vi "Main.vi"(11 "Module Admin":refnum<class "Delacor_lib_QMH_Module Admin.lvclass">) -> ()   [LabVIEW 2020, in "Peek Window.lvlib"]
doc: "This template is based off of the Queued Message Handler design pattern and the Queued Message Handler project template that ships with LabVIEW.\n\nThe main difference is that the queue is private to this module and communication between modules is performed via Broadcast and Request events.\n\nRequest events are wrapped in public API methods and are handled in the Event Handling Loop (EHL) of this VI. Any module can register for Broadcast events sent by this module. The EHL generates messages based on user interface actions.\n\nThe Message Handling Loop (MHL) processes messages generated by the EHL, or by other messages. The messages are string values, so new messages can be added easily to the Message Cases case structure in the MHL. Each message cluster can also provide an optional value for Message Data, which is a variant that can be converted to whatever message-specific data is required.\n_____\nBased on Delacor QMH Project Template 5.0.0.82."
uses:
  Peek Window.lvlib
  <vilib>/Delacor/Delacor QMH/Libraries/Module Admin_class/Delacor_lib_QMH_Module Admin.lvclass
  MHL Data Cluster.ctl
  Open Diagram Argument--cluster.ctl
  EHL Data Cluster.ctl
  Active VI Cluster.ctl
  <vilib>/Delacor/Delacor QMH/Libraries/Message Queue_class/Delacor_lib_QMH_Message Queue.lvclass/Delacor_lib_QMH_Message Queue.ctl
  Stop Argument--cluster.ctl
  <vilib>/Delacor/Delacor QMH/Libraries/Module Admin_class/Delacor_lib_QMH_Module Admin.lvclass/Delacor_lib_QMH_Module Admin.ctl
  Invalid Selection Argument--cluster.ctl
  <vilib>/Delacor/Delacor QMH/Libraries/Message Queue_class/Delacor_lib_QMH_Enqueue Message (Single).vi
  <vilib>/Delacor/Delacor QMH/Libraries/Module Admin_class/Delacor_lib_QMH_Get External Launch.vi
  <vilib>/Utility/error.llb/Error Cluster From Error Code.vi
  <vilib>/ErrorRing/Error Ring.xnode
  <vilib>/Delacor/Delacor QMH/Libraries/Message Queue_class/Delacor_lib_QMH_Message Queue.lvclass
panel:
  in  "File Open":bool
  in  "Previous":bool
  in  "Pin?":bool
  out "Application":string
  in  "Simulate MHL Error":bool
  in  "Simulate EHL Error":bool
  out "error out":errorcluster
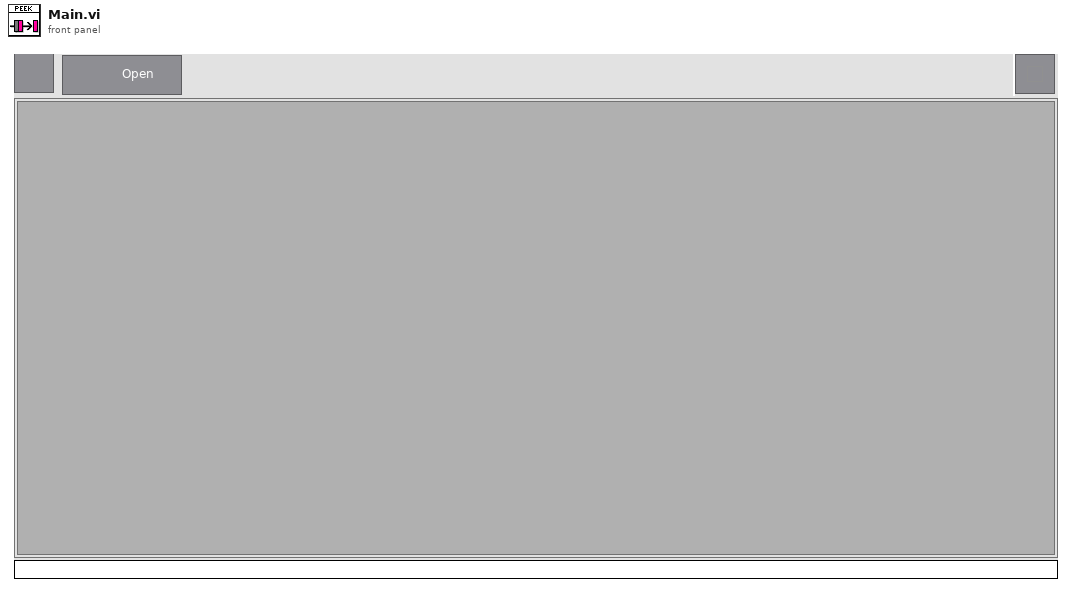
[diagram p1: front panel]
types:
  T1 = typedef "Peek Window.lvlib/EHL Data Cluster.ctl" = cluster{"VI Inserted":string, "Active VI":T2}
  T2 = typedef "Peek Window.lvlib/Active VI Cluster.ctl" = cluster{"App Refnum":refnum<vi>, "VIName":string}
  T3 = typedef "Peek Window.lvlib/MHL Data Cluster.ctl" = cluster{"SubPanel":refnum<vi>, "Call Chain":string[], "Active VI":T4}
  T4 = typedef "Peek Window.lvlib/Open Diagram Argument--cluster.ctl" = cluster{"VI Name":string, "Owning VI Name":string, "App Refnum":refnum<vi>}
  T5 = typedef "Peek Window.lvlib/Request Events--cluster.ctl" = cluster{"Stop Module":refnum<user-event>, "Show Panel":refnum<user-event>, "Hide Panel":refnum<user-event>, "Get Module Execution Status":refnum<user-event>, "Show Diagram":refnum<user-event>, "Open Diagram":refnum<user-event>, "Invalid Selection":refnum<user-event>}
  T6 = enum32{"invalid lock state", "Not Locked", "Locked (No Password)", "Password-protected"}
  T7 = typedef "Peek Window.lvlib/Stop Argument--cluster.ctl" = cluster{"Origin":string, "Exit via Stop Module Req?":bool, "Wait for Module to stop?":bool}
  T8 = typedef "Peek Window.lvlib/Invalid Selection Argument--cluster.ctl" = cluster{"Active VI":string}
  T9 = enum32{"Invalid", "Standard", "Closed", "Hidden", "Minimized", "Maximized"}
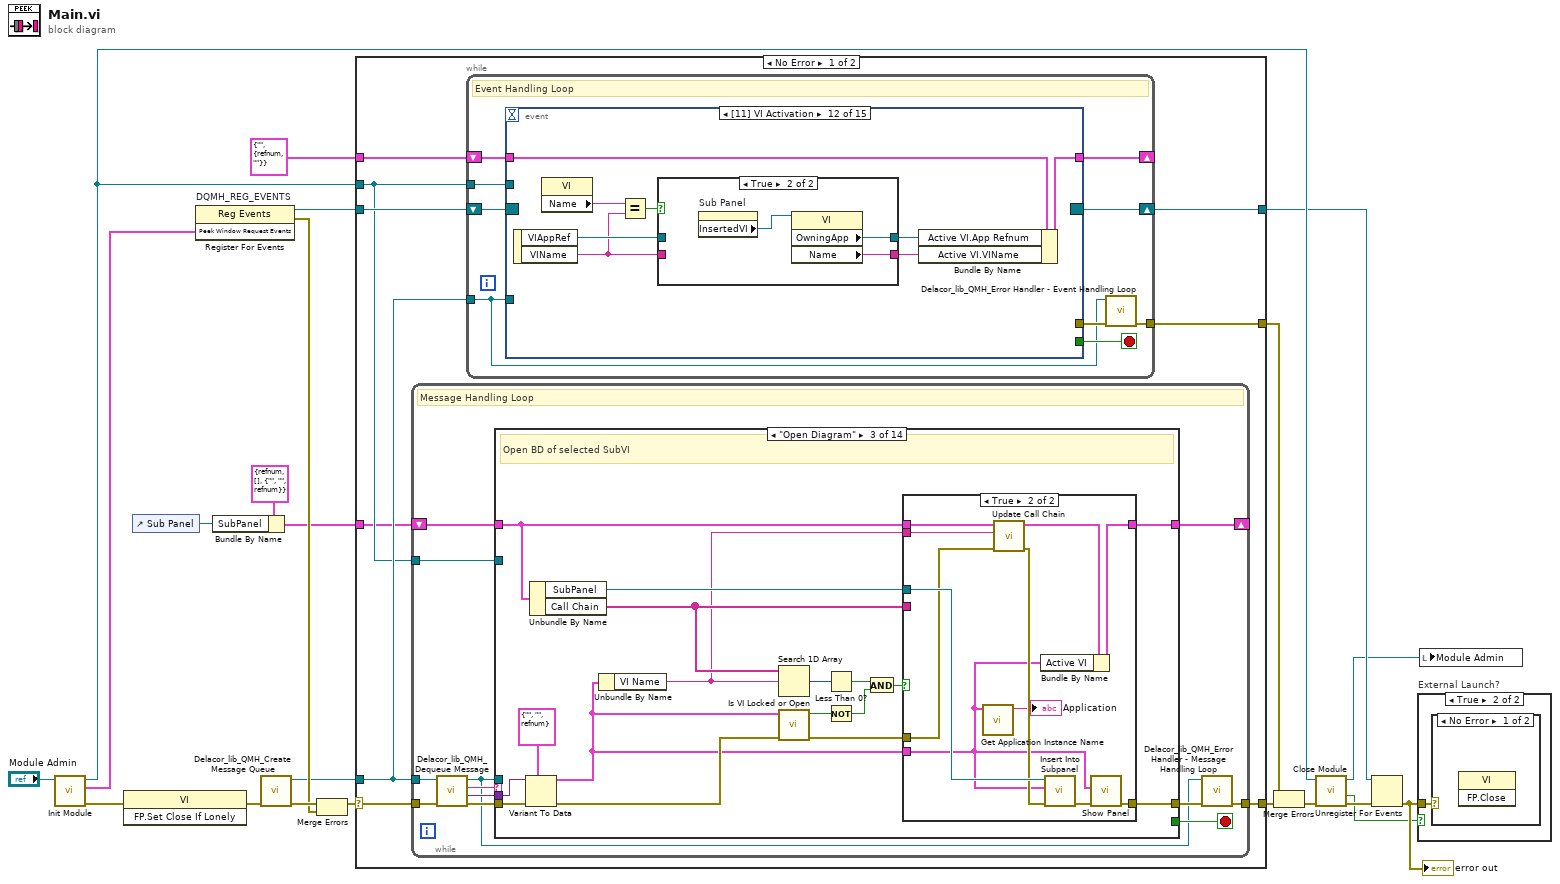
[diagram p0: block diagram]
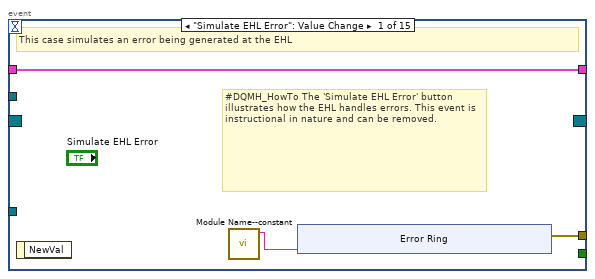
[diagram p2: hidden frame]
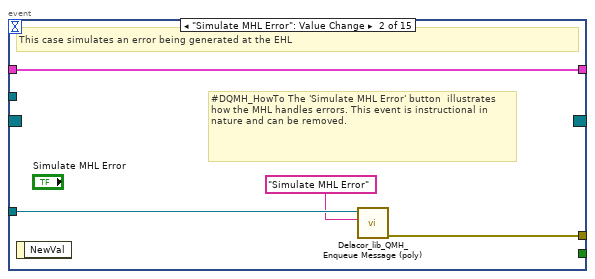
[diagram p3: hidden frame]
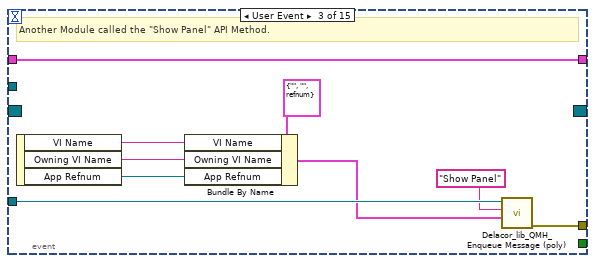
[diagram p4: hidden frame]
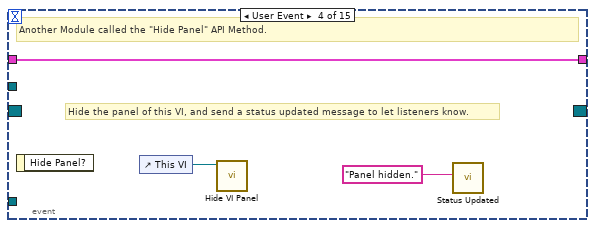
[diagram p5: hidden frame]
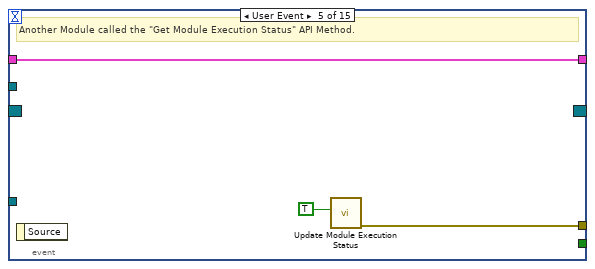
[diagram p6: hidden frame]
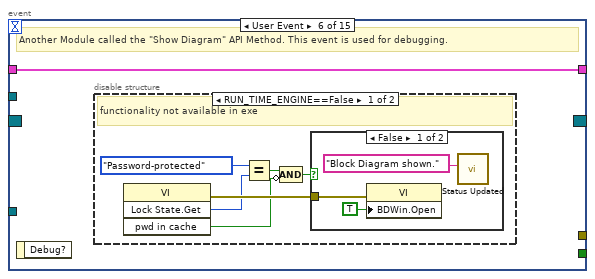
[diagram p7: hidden frame]
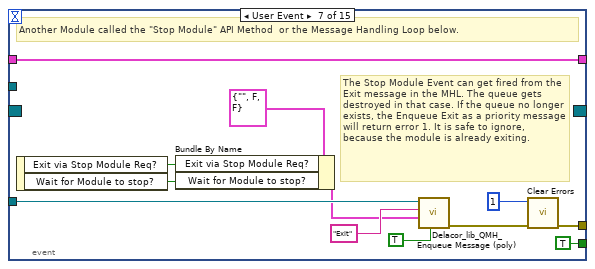
[diagram p10: hidden frame]
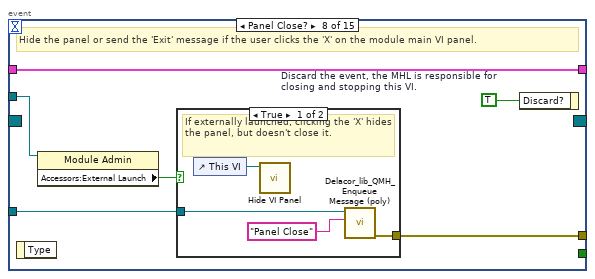
[diagram p11: hidden frame]
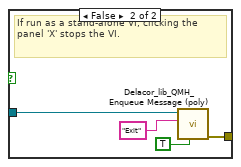
[diagram p12: hidden frame]
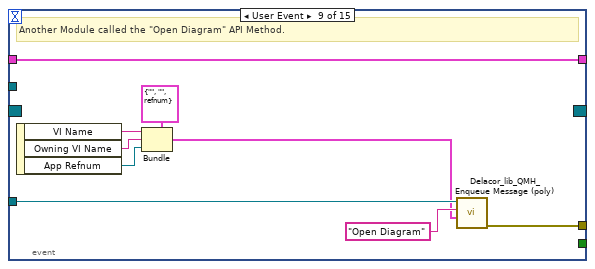
[diagram p13: hidden frame]
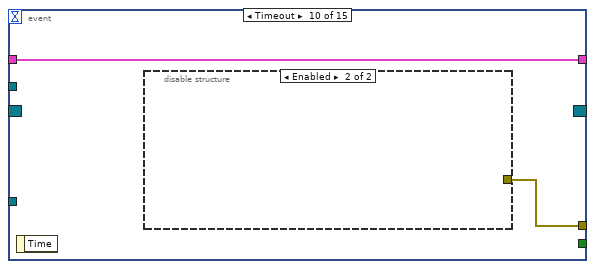
[diagram p14: hidden frame]
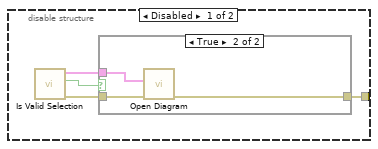
[diagram p15: hidden frame]
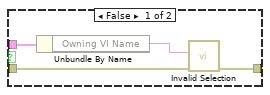
[diagram p16: hidden frame]
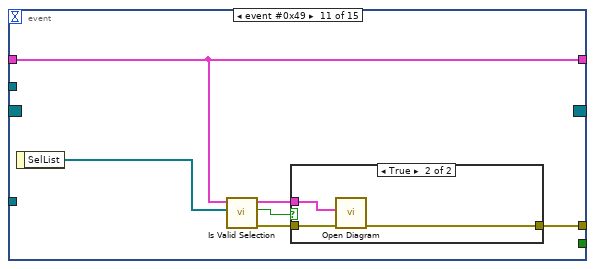
[diagram p17: hidden frame]
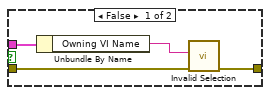
[diagram p18: hidden frame]
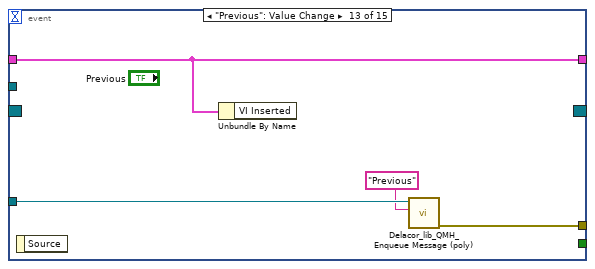
[diagram p20: hidden frame]
diagram:
  n1 = call "Init Module.vi"("Singleton Module Admin in"="Module Admin") -> ("error out"=w2:errorcluster, "Peek Window Request Events"=w11:T5, "Singleton Module Admin out"=w14:refnum<class "Delacor_lib_QMH_Module Admin.lvclass">)  [unwired: 8 in]
  n2 = invoke class="VI" method="FP.Set Close If Lonely"(error in=w2) -> (error out=w1:errorcluster)  [unwired: 2 in, 2 out]
  n3 = control-ref of="Sub Panel"() -> (w4:refnum<vi>)
  n4 = register-events "DQMH_REG_EVENTS"(w11) -> (reference out=w12:refnum<event-registration>, error out=w15:errorcluster)  [unwired: 2 in]
  n5 = Bundle By Name(cluster=T3 {"SubPanel"=refnum, "Call Chain"=[], "Active VI"={"VI Name"="", "Owning VI Name"="", "App Refnum"=refnum}} ("Data Cluster"), "SubPanel"=w4) -> (w5:T3)
  n6 = call <vilib>:"Delacor_lib_QMH_Create Message Queue.vi"("error in (no error)"=w1) -> ("error out"=w17:errorcluster, "Message Queue"=w10:refnum<class "Delacor_lib_QMH_Message Queue.lvclass">)  [unwired: 9 in]
  n7 = Merge Errors(w17, w15) -> (w16:errorcluster)
  n8 = case shown="No Error" w16 {
    selector: w16 -> [w29 w392]
    tunnel: [w31 w391] -> w22
    tunnel: [w28 w397] -> w13
    tunnel: w12 -> [w27 w397]
    tunnel: w10 -> [w26 w390]
    tunnel: [w30 _] -> w20
    tunnel: w14 -> [w25 w393]
    tunnel: w5 -> [w24 _]
    tunnel: T1 {"VI Inserted"="", "Active VI"={"App Refnum"=refnum, "VIName"=""}} ("Data") -> [w23 _]
    frame No Error {
      n9 = while {
        tunnel: w26 -> [w172]
        shift-right: [w169] -> _
        shift-left: w24 -> [w176]
        tunnel: w29 -> [w179]
        tunnel: [w177] -> w31
        tunnel: w25 -> [w170]
        stop <- w175 stop-if-true
        # "Message Handling Loop"
        n10 = call-dynamic "Delacor_lib_QMH_Dequeue Message.vi"("error in (no error)"=w179, "Message Queue in"=w172) -> ("error out"=w178:errorcluster, "Message Data"=w173:variant, "Message"=w174:string, "Message Queue out"=w171:refnum<class "Delacor_lib_QMH_Message Queue.lvclass">)  [unwired: 6 in]
        n11 = case "DQMH_MESSAGE_CASES" shown="\"Open Diagram\"" w174 {
          selector: w174 -> [_ _ _ _ _ _ _ _ _ _ _ _ _ w377]
          tunnel: w171 -> [_ _ _ _ _ _ _ _ _ _ _ w347 w369 _]
          tunnel: w178 -> [w195 w199 w216 w233 w262 w279 w302 w317 w329 w331 w336 w354 w375 w379]
          tunnel: [w193 w199 w213 w238 w257 w280 w302 w308 w328 w331 w335 w350 w372 w380] -> w180
          tunnel: w176 -> [w184 w198 w210 w236 w267 w269 w301 w304 w327 w330 w333 w349 w368 w378]
          tunnel: [w184 w198 w211 w237 w266 w270 w300 w303 w327 w330 w333 w349 w368 w378] -> w169
          tunnel: [_ _ _ _ _ _ _ _ _ _ _ _ w367 _] -> w175
          tunnel: w173 -> [_ _ w215 _ _ w276 _ w316 _ _ _ w348 w366 _]
          tunnel: w170 -> [w185 _ _ _ _ _ _ _ _ _ _ w346 w361 _]
          frame "Initialize" {
            # "#CodeNeeded - Initialize the appearance of the front panel."
            # "#CodeNeeded - Initialize your state data here."
            # "Initialize - Any operation that needs to be done before the module can receive messages. Synchronize Caller Events.vi will inform Start Module.vi that the module has launched and is ready to receive messages. Module Did Init.vi will broadcast that the module initialized."
            n12 = call "Synchronize Caller Events.vi"("error in (no error)"=w195, "Singleton Module Admin in"=w185) -> ("error out"=w194:errorcluster, "Singleton Module Admin out"=w181:refnum<class "Delacor_lib_QMH_Module Admin.lvclass">)  [unwired: 8 in]
            n13 = property on="Property Node" class="Module Admin"(reference=w181) -> ("Accessors:External Launch"=w189:bool)  [unwired: 1 in, 2 out]
            n14 = Select(t=T9."Hidden" ("State"), s=w189, f=T9."Standard" ("State")) -> (s? t:f=w186:T9)
            n15 = call "Module Name--constant.vi"() -> ("Module Name"=w192:string)  [unwired: 11 in]
            n16 = property on="Property Node" class="VI"("Front Panel.Title"=w192) -> (reference out=w191:refnum<vi>, error out=w197:errorcluster)  [unwired: 2 in]
            n17 = call "Module Name--constant.vi"() -> ("Module Name"=w182:string)  [unwired: 11 in]
            n18 = invoke on="Invoke Node" class="VI" method="FP.Open"(reference=w191, error in=w197, "State"=w186) -> (reference out=w190:refnum<vi>, error out=w196:errorcluster)  [unwired: 2 in, 3 out]
            n19 = call "Module Did Init.vi"("error in (no error)"=w194, "Initialized?"=TRUE, "Origin"=w182) -> ("error out"=w193:errorcluster)  [unwired: 8 in]
            n20 = invoke on="Invoke Node" class="VI" method="FP.Center"(reference=w190, error in=w196) -> ()  [unwired: 1 in, 3 out]
          }
          frame "--- Module Specific ---" {
            # "Separator -- The following cases handle messages specific to this Module."
          }
          frame "Open Diagram" {
            # "Open BD of selected SubVI"
            n21 = Variant To Data(error in=w216, type=T4 {"VI Name"="", "Owning VI Name"="", "App Refnum"=refnum} ("Open Diagram Argument"), Variant=w215) -> (data=w200:T4, error out=w204:errorcluster)
            n22 = Unbundle By Name(w210) -> ("SubPanel"=w208:refnum<vi>, "Call Chain"=w209:string[])
            n23 = Unbundle By Name(w200) -> ("VI Name"=w201:string)
            n24 = Search 1D Array(1D array=w209, element=w201) -> (index of element=w212:i32)  [unwired: 1 in]
            n25 = call "Is VI Locked or Open.vi"("Error In"=w204, "VI Info"=w200) -> ("Error Out"=w203:errorcluster, "Locked or Open?"=w206:bool)  [unwired: 8 in]
            n26 = Less Than 0?(x=w212) -> (x < 0?=w207:bool)
            n27 = Not(x=w206) -> (.not. x?=w205:bool)
            n28 = And(x=w207, y=w205) -> (x .and. y?=w202:bool)
            n29 = case shown="True" w202 {
              tunnel: [w218 w224] -> w213
              tunnel: w203 -> [w218 w227]
              tunnel: w201 -> [_ w223]
              tunnel: [w217 w221] -> w211
              tunnel: w210 -> [w217 w228]
              tunnel: w209 -> [_ _]
              tunnel: w208 -> [_ w229]
              tunnel: w200 -> [_ w219]
              frame False {
              }
              frame True {
                n30 = call "Get Application Instance Name.vi"("Active Components"=w219) -> ("Name"=→"Application":string)  [unwired: 10 in]
                n31 = call "Update Call Chain.vi"("error in (no error)"=w227, "VI Name"=w223, "Data Cluster in"=w228) -> ("error out"=w226:errorcluster, "Data Cluster out"=w222:T3)  [unwired: 7 in]
                n32 = Bundle By Name(cluster=w222, "Active VI"=w219) -> (w221:T3)
                n33 = call "Insert Into Subpanel.vi"("error in (no error)"=w226, "Active Components"=w219, "SubPanel in"=w229) -> ("error out"=w225:errorcluster)  [unwired: 7 in, 1 out]
                n34 = call "Show Panel.vi"("error in (no error)"=w225, "Open Diagram Argument"=w219) -> ("error out"=w224:errorcluster)  [unwired: 9 in]
              }
            }
          }
          frame "Previous" {
            # "Open BD of previous SubVI"
            n35 = Unbundle By Name(w236) -> ("Call Chain"=w235:string[], "Active VI"=w231:T4, "SubPanel"=w230:refnum<vi>)
            n36 = Delete From Array(array=w235) -> (array with subset deleted=w234:string[])  [unwired: 2 in, 1 out]
            n37 = Empty Array?(array=w234) -> (empty?=w232:bool)
            n38 = case shown="False" w232 {
              tunnel: [w243 w250] -> w238
              tunnel: [w247 w251] -> w237
              tunnel: w236 -> [w249 w251]
              tunnel: w234 -> [w246 _]
              tunnel: w233 -> [w248 w250]
              tunnel: w230 -> [w239 _]
              tunnel: w231 -> [w241 _]
              frame False {
                n39 = Delete From Array "Replace showing VI\nwith most recent in\ncall chain"(array=w246) -> (deleted portion=w242:string)  [unwired: 2 in, 1 out]
                n40 = Bundle By Name(cluster=w241, "VI Name"=w242) -> (w240:T4)
                n41 = control-ref of="This VI"() -> (w245:refnum<vi>)
                n42 = Bundle By Name(cluster=w249, "Call Chain"=w246) -> (w247:T3)
                n43 = call "Insert Into Subpanel.vi"("error in (no error)"=w248, "Active Components"=w240, "SubPanel in"=w239) -> ("error out"=w244:errorcluster)  [unwired: 7 in, 1 out]
                n44 = call "Position Peek Window.vi"("Error In"=w244, "Subpanel"=w239, "Active Components"=w240, "PeekVI Reference"=w245) -> ("error out"=w243:errorcluster)  [unwired: 7 in]
              }
              frame True {
              }
            }
          }
          frame "File Open" {
            # "Open VI in Current Window"
            n45 = Unbundle By Name(w267) -> ("Active VI.App Refnum"=w252:refnum<vi>, "Call Chain"=w264:string[], "SubPanel"=w261:refnum<vi>)
            n46 = invoke class="SubPnl" method="Remove VI"(reference=w261, error in=w262) -> (error out=w256:errorcluster)  [unwired: 1 in, 2 out]
            n47 = property class="VI"(error in=w256, "FP.State"=T9."Hidden" ("Front Panel Window:State")) -> (error out=w255:errorcluster)  [unwired: 1 in, 1 out]
            n48 = Delete From Array(array=w264) -> (deleted portion=w263:string)  [unwired: 2 in, 1 out]
            n49 = Open VI Reference(application reference (local)=w252, vi path=w263, error in (no error)=w255) -> (vi reference=w259:refnum<vi>, error out=w260:errorcluster)  [unwired: 3 in]
            n50 = Bundle By Name(cluster=w267, "Call Chain"=string[] []) -> (w266:T3)
            n51 = property class="VI"(reference=w259, error in=w260, "BDWin.Open"=TRUE ("Block Diagram Window:Open"), "FP.State"=T9."Minimized" ("Front Panel Window:State")) -> (error out=w257:errorcluster)  [unwired: 1 out]
          }
          frame "Show Panel" {
            n52 = Variant To Data(error in=w279, type=T4 {"VI Name"="", "Owning VI Name"="", "App Refnum"=refnum} ("Open Diagram Argument"), Variant=w276) -> (data=w268:T4, error out=w277:errorcluster)
            n53 = Bundle By Name(cluster=w269, "Active VI"=w268) -> (w270:T3)
            n54 = Unbundle By Name(w270) -> ("Call Chain"=w273:string[], "SubPanel"=w271:refnum<vi>)
            n55 = control-ref of="This VI"() -> (w275:refnum<vi>)
            n56 = Empty Array?(array=w273) -> (empty?=w272:bool)
            n57 = case shown="False" w272 {
              tunnel: [w286 w298] -> w280
              tunnel: w277 -> [w287 w298]
              tunnel: "Pin?" -> [w285 _]
              tunnel: w268 -> [w283 _]
              tunnel: w275 -> [w284 _]
              tunnel: w273 -> [w282 _]
              tunnel: w271 -> [w281 _]
              frame False {
                # "Call Chain not empty"
                n58 = case shown="False" w285 {
                  tunnel: w287 -> [w294 w297]
                  tunnel: [w295 w297] -> w286
                  tunnel: w284 -> [w293 _]
                  tunnel: w283 -> [w289 _]
                  tunnel: w282 -> [w291 _]
                  tunnel: w281 -> [w288 _]
                  frame False {
                    # "Not pinned"
                    n59 = Delete From Array "Replace showing VI\nwith most recent in\ncall chain"(array=w291) -> (deleted portion=w292:string)  [unwired: 2 in, 1 out]
                    n60 = Bundle By Name(cluster=w289, "VI Name"=w292) -> (w290:T4)
                    n61 = call "Position Peek Window.vi"("Error In"=w294, "Subpanel"=w288, "Active Components"=w290, "PeekVI Reference"=w293) -> ("error out"=w295:errorcluster)  [unwired: 7 in]
                  }
                  frame True {
                    # "Pinned"
                    n62 = property class="VI"("FP.State"=T9."Standard" ("Front Panel Window:State")) -> ()  [unwired: 2 in, 2 out]
                  }
                }
              }
              frame True {
                # "Nothing in Call Chain"
              }
            }
          }
          frame "Panel Close" {
            n63 = Bundle By Name(cluster=w301, "Call Chain"=string[] []) -> (w300:T3)
          }
          frame "Invalid Selection" {
            n64 = Variant To Data(error in=w317, type=T8 {"Active VI"=""} ("Invalid Selection Argument"), Variant=w316) -> (data=w314:T8, error out=w309:errorcluster)
            n65 = Unbundle By Name(w304) -> ("Call Chain"=w313:string[])
            n66 = property class="VI"() -> ("Name"=w312:string)  [unwired: 2 in, 2 out]
            n67 = Unbundle By Name(w314) -> ("Active VI"=w310:string)
            n68 = Build Array (concatenate)(w313, w312, "VI Hierarchy") -> (w311:string[])
            n69 = Search 1D Array(1D array=w311, element=w310) -> (index of element=w307:i32)  [unwired: 1 in]
            n70 = Less Than 0?(x=w307) -> (x < 0?=w306:bool)
            n71 = case shown="True" w306 {
              tunnel: w309 -> [w319 w321]
              tunnel: [w319 w320] -> w308
              tunnel: w304 -> [w318 w323]
              tunnel: [w318 w325] -> w303
              frame False {
              }
              frame True {
                n72 = Unbundle By Name(w323) -> ("SubPanel"=w322:refnum<vi>)
                n73 = invoke class="SubPnl" method="Remove VI"(reference=w322, error in=w321) -> (error out=w320:errorcluster)  [unwired: 1 in, 2 out]
                n74 = property class="VI"("FP.State"=T9."Hidden" ("Front Panel Window:State")) -> ()  [unwired: 2 in, 2 out]
                n75 = Bundle By Name(cluster=w323, "Call Chain"=string[] []) -> (w325:T3)
              }
            }
          }
          frame "---Copy This Frame---" {
            # "Duplicate this frame when creating new messages.  Change this comment in the duplicated frame to describe this message."
            n76 = Merge Errors(w329) -> (w328:errorcluster)
          }
          frame "--- Exit and Error Handling---" {
            # "Separator - The following cases handle errors and exit messages."
          }
          frame "Simulate MHL Error" {
            # "#DQMH_HowTo The 'Simulate MHL Error' button  illustrates how the MHL handles errors. This event is instructional in nature and can be removed."
            # "Simulate an error occurring at the MHL"
            n77 = call "Module Name--constant.vi"() -> ("Module Name"=w332:string)  [unwired: 11 in]
            n78 = xnode "Error Ring"("parameter 0"=w332) -> ("error out"=w334:errorcluster)
            n79 = Merge Errors(w336, w334) -> (w335:errorcluster)
          }
          frame "Error" {
            # "#CodeRecommended - If you ever change the name of this \"Error\" message, you'll need to update the name in the Check Loop Error.vi as well."
            # "#CodeRecommended - If the module is running in standalone mode (External Launch = FALSE), this code will pop up an error dialog and call the 'Exit' message if an error occurs. Add more fine-grained error handling here."
            # "Error - Check the error message data and respond accordingly. This message is sent by the \"Error Handler\" VIs at the end of each loop in this application."
            n80 = property on="Property Node" class="Module Admin"(reference=w346) -> ("Accessors:External Launch"=w345:bool)  [unwired: 1 in, 2 out]
            n81 = Variant To Data(error in=w354, type=errorcluster {"status"=FALSE, "code"=0, "source"=""} ("error constant"), Variant=w348) -> (data=w355:errorcluster, error out=w352:errorcluster)
            n82 = call "Module Name--constant.vi"() -> ("Module Name"=w344:string)  [unwired: 11 in]
            n83 = call "Error Reported.vi"("Additional Information"=w344, "Error"=w355) -> ()  [unwired: 9 in, 1 out]
            n84 = case shown="False" w345 {
              tunnel: [w360 _] -> w351
              tunnel: w347 -> [w358 _]
              tunnel: w355 -> [w359 _]
              frame False {
                # "If the module is running standalone, then pop up an error dialog and call the \"Exit\" message."
                n85 = call <vilib>:"Simple Error Handler.vi"("error in (no error)"=w359) -> ()  [unwired: 4 in, 5 out]
                n86 = call-poly <vilib>:"Delacor_lib_QMH_Enqueue Message (poly).vi"("Priority Message? (F)"=TRUE, "Message"="Exit", "Message Queue in"=w358) -> ("error out"=w360:errorcluster)  [unwired: 7 in, 1 out]
              }
              frame True {
                # "If the module was launched externally, calling the Error Reported broadcast VI is the only action performed by the \"Error\" message. The module's caller can then process the error appropriately."
              }
            }
            n87 = Merge Errors(w352, w351) -> (w350:errorcluster)
            n88 = local write "error out"(w350) -> ()
          }
          frame "Exit" {
            w365 = 91  # 91: not all Exit messages will have an argument
            w367 = TRUE  # Stop the VI
            # "Release the message queue reference"
            # "#CodeNeeded - Add any required cleanup code here"
            # "Exit - Exit the application."
            n89 = Variant To Data(error in=w375, type=T7 {"Origin"="", "Exit via Stop Module Req?"=FALSE, "Wait for Module to stop?"=FALSE} ("Stop Argument"), Variant=w366) -> (data=w363:T7, error out=w371:errorcluster)
            n90 = call <vilib>:"Clear Errors.vi"("error in (no error)"=w371, "specific error code to clear (0: all)"=w365) -> ("error out"=w374:errorcluster)  [unwired: 4 in, 1 out]
            n91 = control-ref of="This VI"() -> (w362:refnum<vi>)
            n92 = call-dynamic "Delacor_lib_QMH_Release Message Queue.vi"("error in (no error)"=w374, "Message Queue"=w369) -> ("error out"=w373:errorcluster)  [unwired: 9 in]
            n93 = call "Handle Exit.vi"("Stop Argument"=w363, "Admin in"=w361, "VI reference"=w362) -> ("error out"=w370:errorcluster)  [unwired: 7 in, 1 out]
            n94 = Merge Errors(w373, w370) -> (w372:errorcluster)
          }
          frame Default {
            # "'Default' case only runs if there is a message that isn't defined in any of the other cases.  Output a programming error."
            n95 = call "Module Name--constant.vi"() -> ("Module Name"=w376:string)  [unwired: 11 in]
            n96 = xnode "Error Ring"("parameter 0"=w377, "parameter 1"=w376) -> ("error out"=w381:errorcluster)
            n97 = Merge Errors(w379, w381) -> (w380:errorcluster)
          }
        }
        n98 = call-dynamic "Delacor_lib_QMH_Error Handler - Message Handling Loop.vi"("error in (no error)"=w180, "Message Queue in"=w171) -> ("dup error in"=w177:errorcluster)  [unwired: 8 in, 1 out]
      }
      n99 = while {
        tunnel: w26 -> [w34]
        shift-right: [w37] -> w28
        shift-left: w27 -> [w38]
        tunnel: [w39] -> w30
        tunnel: w25 -> [w35]
        shift-right: [w32] -> _
        shift-left: w23 -> [w33]
        stop <- w36 stop-if-true
        # "Event Handling Loop"
        n100 = event "DQMH_EVENT_MAIN" shown="[11] VI Activation" {
          selector: w38 -> [_ _ _ _ _ _ _ _ _ _ _ _ _ _ _]
          dyn-events: [_ _ _ _ _ _ _ _ _ _ _ _ _ _ _] -> w37
          timeout: _ -> [_ _ _ _ _ _ _ _ _ _ _ _ _ _ _]
          tunnel: [_ _ _ _ _ _ TRUE ("Discard?") _ _ _ _ _ _ _ _] -> w36
          tunnel: w34 -> [_ w53 w62 _ _ _ w87 w95 w114 _ _ _ w157 w160 w167]
          tunnel: [w43 w54 w61 _ w69 _ w90 w97 w109 w115 w131 _ w156 w159 w162] -> w40
          tunnel: w35 -> [_ _ _ _ _ _ _ w94 _ _ _ _ _ _ _]
          tunnel: w33 -> [w41 w51 w63 w64 w67 w70 w80 w92 w108 w116 w129 w147 w154 w161 w168]
          tunnel: [w41 w51 w63 w64 w67 w70 w80 w92 w108 w116 w129 w148 w154 w161 w168] -> w32
          event "Simulate EHL Error": Value Change {
            # "#DQMH_HowTo The 'Simulate EHL Error' button  illustrates how the EHL handles errors. This event is instructional in nature and can be removed."
            # "This case simulates an error being generated at the EHL"
            n101 = event-data() -> ()  [unwired: 1 in, 1 out]
            n102 = call "Module Name--constant.vi"() -> ("Module Name"=w42:string)  [unwired: 11 in]
            n103 = xnode "Error Ring"("parameter 0"=w42) -> ("error out"=w43:errorcluster)
          }
          event "Simulate MHL Error": Value Change {
            # "#DQMH_HowTo The 'Simulate MHL Error' button  illustrates how the MHL handles errors. This event is instructional in nature and can be removed."
            # "This case simulates an error being generated at the EHL"
            n104 = event-data() -> ()  [unwired: 1 in, 1 out]
            n105 = call-poly <vilib>:"Delacor_lib_QMH_Enqueue Message (poly).vi"("Message"="Simulate MHL Error", "Message Queue in"=w53) -> ("error out"=w54:errorcluster)  [unwired: 8 in, 1 out]
          }
          event User Event {
            # "Another Module called the \"Show Panel\" API Method."
            n106 = event-data() -> ("VI Name"=w58:string, "Owning VI Name"=w56:string, "App Refnum"=w55:refnum<vi>)  [unwired: 1 in]
            n107 = Bundle By Name(cluster=T4 {"VI Name"="", "Owning VI Name"="", "App Refnum"=refnum} ("Open Diagram Argument"), "VI Name"=w58, "Owning VI Name"=w56, "App Refnum"=w55) -> (w57:T4)
            n108 = call-poly <vilib>:"Delacor_lib_QMH_Enqueue Message (poly).vi"("Message Data"=w57, "Message"="Show Panel", "Message Queue in"=w62) -> ("error out"=w61:errorcluster)  [unwired: 7 in, 1 out]
          }
          event User Event {
            # "Hide the panel of this VI, and send a status updated message to let listeners know."
            # "Another Module called the \"Hide Panel\" API Method."
            n109 = event-data() -> ()  [unwired: 1 in, 1 out]
            n110 = control-ref of="This VI"() -> (w66:refnum<vi>)
            n111 = call "Hide VI Panel.vi"("VI"=w66) -> ()  [unwired: 10 in, 1 out]
            n112 = call "Status Updated.vi"("Status"="Panel hidden." ("format string")) -> ()  [unwired: 10 in, 1 out]
          }
          event User Event {
            # "Another Module called the \"Get Module Execution Status\" API Method."
            n113 = event-data() -> ()  [unwired: 1 in, 1 out]
            n114 = call "Update Module Execution Status.vi"("Running?"=TRUE) -> ("error out"=w69:errorcluster)  [unwired: 10 in]
          }
          event User Event {
            # "Another Module called the \"Show Diagram\" API Method. This event is used for debugging."
            n115 = event-data() -> ()  [unwired: 1 in, 1 out]
            n116 = disable-structure shown="RUN_TIME_ENGINE==False" {
              frame condition #0 (active) {
                # "functionality not available in exe"
                n117 = invoke on="Invoke Node" class="VI" method="Lock State.Get"() -> (error out=w76:errorcluster, "Get Lock State"=w75:T6, "pwd in cache"=w72:bool)  [unwired: 4 in, 1 out]
                n118 = Equal?(x=T6."Password-protected", y=w75) -> (x = y?=w73:bool)
                n119 = Compound Arithmetic op=AND(w73, invert w72) -> (w71:bool)
                n120 = case shown="False" w71 {
                  tunnel: w76 -> [w79 _]
                  frame False {
                    n121 = property on="Property Node" class="VI"(error in=w79, "BDWin.Open"=TRUE ("Block Diagram Window:Open")) -> ()  [unwired: 1 in, 2 out]
                    n122 = call "Status Updated.vi"("Status"="Block Diagram shown." ("format string")) -> ()  [unwired: 10 in, 1 out]
                  }
                  frame True {
                    # "Password-protected VI, and the password is not in the cache. Do not show the diagram."
                  }
                }
              }
              frame condition #1 {
              }
            }
          }
          event User Event {
            # "The Stop Module Event can get fired from the Exit message in the MHL. The queue gets destroyed in that case. If the queue no longer exists, the Enqueue Exit as a priority message will return error 1. It is safe to ignore, because the module is already exiting."
            # "Another Module called the \"Stop Module\" API Method  or the Message Handling Loop below."
            n123 = event-data() -> ("Exit via Stop Module Req?"=w83:bool, "Wait for Module to stop?"=w82:bool)  [unwired: 1 in]
            n124 = Bundle By Name(cluster=T7 {"Origin"="", "Exit via Stop Module Req?"=FALSE, "Wait for Module to stop?"=FALSE} ("Stop Argument"), "Exit via Stop Module Req?"=w83, "Wait for Module to stop?"=w82) -> (w81:T7)
            n125 = call-poly <vilib>:"Delacor_lib_QMH_Enqueue Message (poly).vi"("Priority Message? (F)"=TRUE, "Message Data"=w81, "Message"="Exit", "Message Queue in"=w87) -> ("error out"=w91:errorcluster)  [unwired: 6 in, 1 out]
            n126 = call <vilib>:"Clear Errors.vi"("error in (no error)"=w91, "specific error code to clear (0: all)"=1) -> ("error out"=w90:errorcluster)  [unwired: 4 in, 1 out]
          }
          event Panel Close? {
            w96 = TRUE  # Discard the event, the MHL is responsible for closing and stopping this VI.
            # "Hide the panel or send the 'Exit' message if the user clicks the 'X' on the module main VI panel."
            n127 = event-data() -> ()  [unwired: 1 in, 1 out]
            n128 = property on="Property Node" class="Module Admin"(reference=w94) -> ("Accessors:External Launch"=w93:bool)  [unwired: 1 in, 2 out]
            n129 = case shown="True" w93 {
              tunnel: w95 -> [w100 w104]
              tunnel: [w99 w105] -> w97
              frame True {
                # "If externally launched, clicking the 'X' hides the panel, but doesn't close it."
                n130 = control-ref of="This VI"() -> (w101:refnum<vi>)
                n131 = call "Hide VI Panel.vi"("VI"=w101) -> ()  [unwired: 10 in, 1 out]
                n132 = call-poly <vilib>:"Delacor_lib_QMH_Enqueue Message (poly).vi"("Message"="Panel Close", "Message Queue in"=w100) -> ("error out"=w99:errorcluster)  [unwired: 8 in, 1 out]
              }
              frame False {
                # "If run as a stand-alone VI, clicking the panel 'X' stops the VI."
                n133 = call-poly <vilib>:"Delacor_lib_QMH_Enqueue Message (poly).vi"("Priority Message? (F)"=TRUE, "Message"="Exit", "Message Queue in"=w104) -> ("error out"=w105:errorcluster)  [unwired: 7 in, 1 out]
              }
            }
            n134 = event-data ("Event Filter Node")("Discard?"=w96) -> ()  [unwired: 1 in, 1 out]
          }
          event User Event {
            # "Another Module called the \"Open Diagram\" API Method."
            n135 = event-data() -> ("VI Name"=w110:string, "Owning VI Name"=w107:string, "App Refnum"=w106:refnum<vi>)  [unwired: 1 in]
            n136 = Bundle(cluster=T4 {"VI Name"="", "Owning VI Name"="", "App Refnum"=refnum} ("Open Diagram Argument"), "VI Name"=w110, "Owning VI Name"=w107, "App Refnum"=w106) -> (w111:T4)
            n137 = call-poly <vilib>:"Delacor_lib_QMH_Enqueue Message (poly).vi"("Message Data"=w111, "Message"="Open Diagram", "Message Queue in"=w114) -> ("error out"=w109:errorcluster)  [unwired: 7 in, 1 out]
          }
          event Timeout {
            n138 = event-data() -> ()  [unwired: 1 in, 1 out]
            n139 = disable-structure shown="Enabled" {
              disable-tunnel: [w118 _] -> w115
              frame Disabled {
                n140 = call "Is Valid Selection"() -> ("error out"=w120:errorcluster, "Valid Selected?"=w119:bool, "Active Components"=w117:T4)  [unwired: 9 in]
                n141 = case shown="True" w119 {
                  tunnel: w117 -> [w122 w126]
                  tunnel: w120 -> [w124 w125]
                  tunnel: [w123 w127] -> w118
                  frame False {
                    n142 = Unbundle By Name(w122) -> ("Owning VI Name"=w121:string)
                    n143 = call "Invalid Selection.vi"("error in (no error)"=w124, "Active VI"=w121) -> ("error out"=w123:errorcluster)  [unwired: 9 in]
                  }
                  frame True {
                    n144 = call "Open Diagram.vi"("error in (no error)"=w125, "DQMH_ARG"=w126) -> ("error out"=w127:errorcluster)  [unwired: 9 in]
                  }
                }
              }
              frame Enabled {
              }
            }
          }
          event event #0x49 {
            n145 = event-data() -> ("SelList"=w128:refnum<vi>[])  [unwired: 1 in]
            n146 = call "Is Valid Selection"("SelList"=w128, "Data"=w129) -> ("error out"=w133:errorcluster, "Valid Selected?"=w132:bool, "Active Components"=w130:T4)  [unwired: 7 in]
            n147 = case shown="True" w132 {
              tunnel: w130 -> [w135 w139]
              tunnel: w133 -> [w137 w138]
              tunnel: [w136 w140] -> w131
              frame False {
                n148 = Unbundle By Name(w135) -> ("Owning VI Name"=w134:string)
                n149 = call "Invalid Selection.vi"("error in (no error)"=w137, "Active VI"=w134) -> ("error out"=w136:errorcluster)  [unwired: 9 in]
              }
              frame True {
                n150 = call "Open Diagram.vi"("error in (no error)"=w138, "DQMH_ARG"=w139) -> ("error out"=w140:errorcluster)  [unwired: 9 in]
              }
            }
          }
          event VI Activation {
            n151 = event-data() -> ("VIAppRef"=w144:refnum<vi>, "VIName"=w143:string)  [unwired: 1 in]
            n152 = property class="VI"() -> ("Name"=w146:string)  [unwired: 2 in, 2 out]
            n153 = Equal?(x=w146, y=w143) -> (x = y?=w145:bool)
            n154 = case shown="True" w145 {
              tunnel: [w150 w151] -> w141
              tunnel: w144 -> [w150 _]
              tunnel: w143 -> [w149 _]
              tunnel: [w149 w152] -> w142
              frame False {
              }
              frame True {
                n155 = property on="Sub Panel" class="SubPnl"() -> ("InsertedVI"=w153:refnum<vi>)  [unwired: 2 in, 2 out]
                n156 = property class="VI"(reference=w153) -> ("OwningApp"=w151:refnum<vi>, "Name"=w152:string)  [unwired: 1 in, 2 out]
              }
            }
            n157 = Bundle By Name(cluster=w147, "Active VI.App Refnum"=w141, "Active VI.VIName"=w142) -> (w148:T1)
          }
          event "Previous": Value Change {
            n158 = event-data() -> ()  [unwired: 1 in, 1 out]
            n159 = Unbundle By Name(w154) -> ()  [unwired: 1 out]
            n160 = call-poly <vilib>:"Delacor_lib_QMH_Enqueue Message (poly).vi"("Message"="Previous", "Message Queue in"=w157) -> ("error out"=w156:errorcluster)  [unwired: 8 in, 1 out]
          }
          event "File Open": Value Change {
            n161 = event-data() -> ()  [unwired: 1 in, 1 out]
            n162 = call-poly <vilib>:"Delacor_lib_QMH_Enqueue Message (poly).vi"("Message"="File Open", "Message Queue in"=w160) -> ("error out"=w159:errorcluster)  [unwired: 8 in, 1 out]
          }
          event User Event {
            # "Another Module called the \"Invalid Selection\" API Method."
            n163 = event-data() -> ("Active VI"=w163:string)  [unwired: 1 in]
            n164 = Bundle(cluster=T8 {"Active VI"=""} ("Invalid Selection Argument"), "Active VI"=w163) -> (w164:T8)
            n165 = call-poly <vilib>:"Delacor_lib_QMH_Enqueue Message (poly).vi"("Message Data"=w164, "Message"="Invalid Selection", "Message Queue in"=w167) -> ("error out"=w162:errorcluster)  [unwired: 7 in, 1 out]
          }
        }
        n166 = call-dynamic "Delacor_lib_QMH_Error Handler - Event Handling Loop.vi"("error in (no error)"=w40, "Message Queue in"=w34) -> ("dup error in"=w39:errorcluster)  [unwired: 8 in, 1 out]
      }
    }
    frame Error {
      # "Synchronize Caller Events.vi will inform Start Module.vi that the module has launched and will let the code calling Start Module.vi register for broadcasts and would permit the caller receive the broadcast that an error occurred at launch time."
      n167 = call-dynamic "Delacor_lib_QMH_Release Message Queue.vi"("error in (no error)"=w392, "Message Queue"=w390) -> ("error out"=w391:errorcluster)  [unwired: 9 in]
      n168 = call "Synchronize Caller Events.vi"("Singleton Module Admin in"=w393) -> ("error out"=w398:errorcluster)  [unwired: 9 in, 1 out]
      n169 = call "Module Name--constant.vi"() -> ("Module Name"=w396:string)  [unwired: 11 in]
      n170 = Format Into String(format string="An error occurred during initialization. %s is no longer running.", w396) -> (resulting string=w394:string)  [unwired: 2 in, 1 out]
      n171 = Merge Errors(w391, w398) -> (w399:errorcluster)
      n172 = call "Error Reported.vi"("Additional Information"=w394, "Error"=w399) -> ()  [unwired: 9 in, 1 out]
    }
  }
  n173 = Merge Errors(w20, w22) -> (w19:errorcluster)
  n174 = call "Close Module.vi"("error in (no error)"=w19, "Module Admin in"=w14) -> ("error out"=w21:errorcluster, "External Launch"=w7:bool, "Module Admin out"=w8:refnum<class "Delacor_lib_QMH_Module Admin.lvclass">)  [unwired: 7 in]
  n175 = Unregister For Events(event registration refnum=w13, error in=w21) -> (error out=w18:errorcluster)
  "error out" <- w18
  n176 = case "External Launch?" shown="True" w7 {
    tunnel: w18 -> [_ w400]
    frame False {
    }
    frame True {
      n177 = case shown="No Error" w400 {
        frame No Error {
          n178 = invoke on="Invoke Node" class="VI" method="FP.Close"() -> ()  [unwired: 3 in, 3 out]
        }
        frame Error {
          n179 = invoke on="Invoke Node" class="VI" method="FP.Open"("Activate"=TRUE ("Activate?")) -> ()  [unwired: 4 in, 5 out]
        }
      }
    }
  }
  n180 = local write "Module Admin"(w8) -> ()
